vi "Configure Voltage.vi"(8 "error in (no error)":errorcluster, 10 "Voltage":dbl, 11 "E3610x in":refnum<class "E3610x.lvclass">) -> (0 "error out":errorcluster, 3 "E3610x out":refnum<class "E3610x.lvclass">)   [LabVIEW 2020, in "E3610x.lvclass"]
uses:
  E3610x.lvclass
  C:/Sandbox/RF Bench/Source Code/WiSpry Test Framework/Instruments/Instrument.lvclass
  Instrument.lvclass/Instrument.ctl
  E3610x.lvclass/E3610x.ctl
  Instrument.lvclass
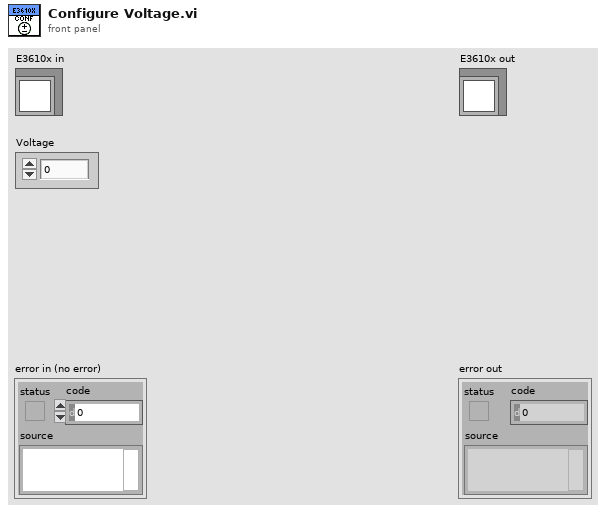
[diagram p1: front panel]
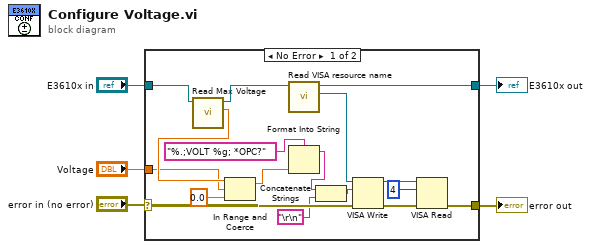
[diagram p0: block diagram]
diagram:
  n1 = case shown="No Error" "error in (no error)" {
    selector: "error in (no error)" -> [w22 w24]
    tunnel: "E3610x in" -> [w11 w23]
    tunnel: "Voltage" -> [w7 _]
    tunnel: [w16 w24] -> w2
    tunnel: [w15 w23] -> w1
    frame No Error {
      n2 = call "Read Max Voltage.vi"("E3610x in"=w11) -> ("Max Voltage"=w9:dbl, "E3610x out"=w10:refnum<class "E3610x.lvclass">)  [unwired: 9 in]
      n3 = In Range and Coerce(upper limit=w9, x=w7, lower limit=0.0) -> (coerced(x)=w6:dbl)  [unwired: 1 out]
      n4 = call "Read VISA resource name.vi"("Instrument in"=w10) -> ("VISA resource name"=w21:refnum<visa-resource-name>, "Instrument out"=w15:refnum<class "E3610x.lvclass">)  [unwired: 9 in]
      n5 = Format Into String(format string="%.;VOLT %g; *OPC?" ("initial string"), w6) -> (resulting string=w20:string)  [unwired: 2 in, 1 out]
      n6 = Concatenate Strings(w20, "\r\n") -> (w14:string)
      n7 = VISA Write(VISA resource name=w21, write buffer=w14, error in (no error)=w22) -> (VISA resource name out=w18:refnum<visa-resource-name>, error out=w19:errorcluster)  [unwired: 1 out]
      n8 = VISA Read(VISA resource name=w18, byte count=u32 4, error in (no error)=w19) -> (error out=w16:errorcluster)  [unwired: 3 out]
    }
    frame Error {
    }
  }
  "error out" <- w2
  "E3610x out" <- w1
